vi "timed relay control.vi"(8 "reverse time":u32=350, 9 "start reverse":bool, 10 "start forward":bool, 11 "forward time":u32=350) -> (1 "complete":bool, 3 "output to relay":T1)   [LabVIEW 2016]
uses:
  <vilib>/Rock Robotics/WPI/Relay/WPI_RelayValue.ctl
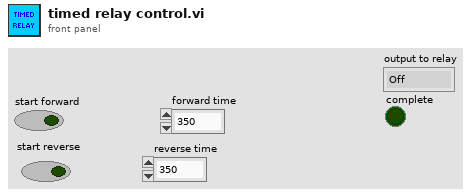
[diagram p1: front panel]
types:
  T1 = typedef "WPI_RelayValue.ctl" = enum16{"Off", "On", "Forward", "Reverse"}
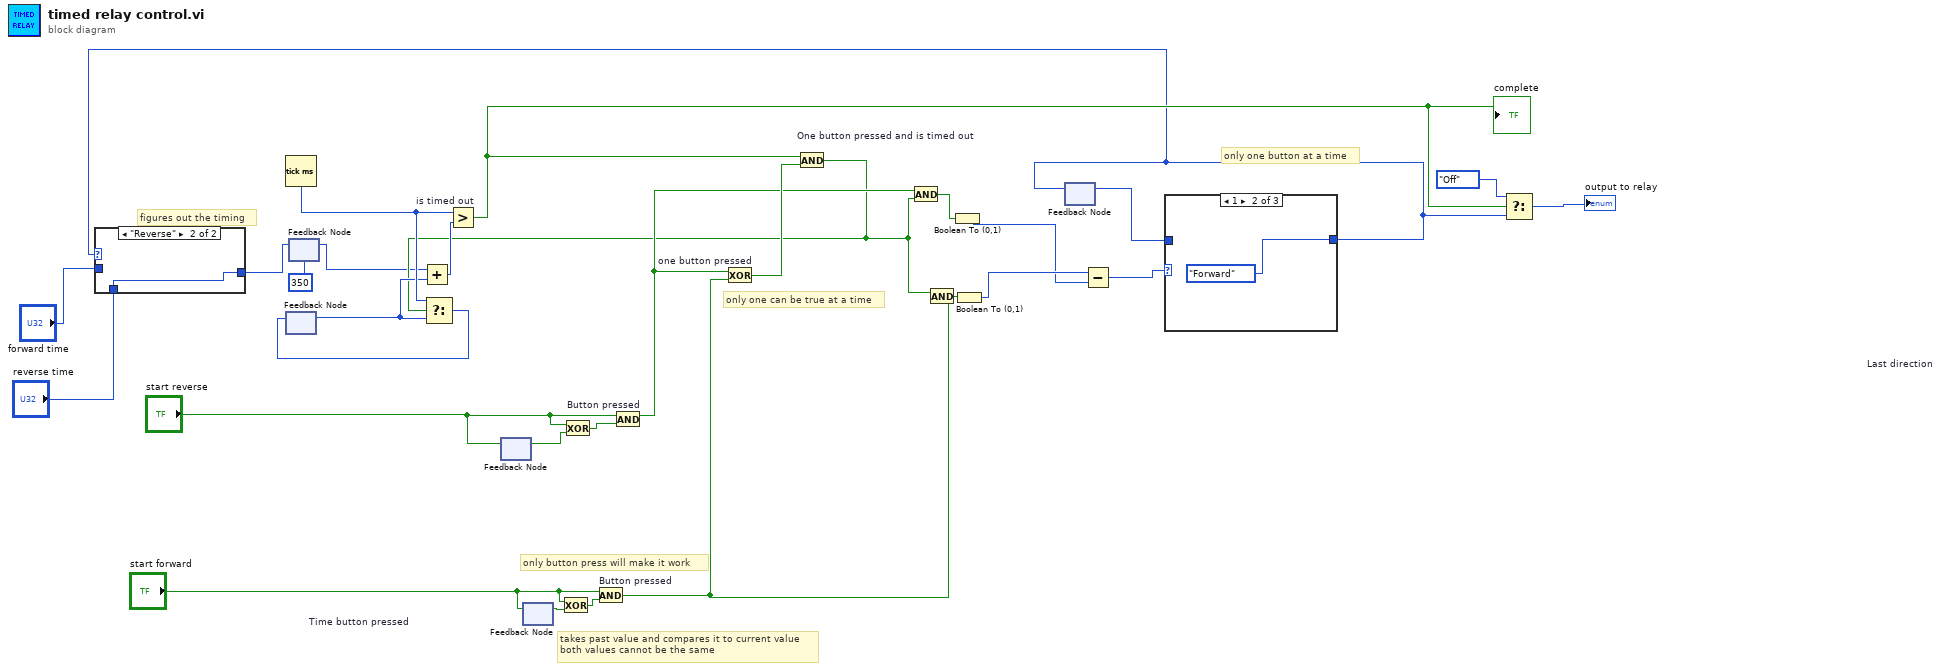
[diagram p0: block diagram]
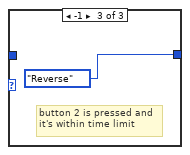
[diagram p4: hidden frame]
diagram:
  # "figures out the timing"
  # "takes past value and compares it to current value\nboth values cannot be the same"
  # "only one button at a time"
  # "only button press will make it work"
  # "only one can be true at a time"
  n1 = Tick Count (ms)() -> (millisecond timer value=w29:u32)
  n2 = feedback #1 "Time button pressed"() -> (w14:u32)  [unwired: 1 in]
  n3 = feedback #2(u32 350 ("y")) -> (w8:u32)
  n4 = Add(x=w8, y=w14) -> (x+y=w27:u32)
  n5 = Greater? "is timed out"(x=w29, y=w27) -> (0:w18:bool)
  "complete" <- w18
  n6 = feedback #3() -> (w25:bool)  [unwired: 1 in]
  n7 = feedback-in #3("start reverse") -> ()
  n8 = feedback #4() -> (w6:bool)  [unwired: 1 in]
  n9 = feedback-in #4("start forward") -> ()
  n10 = Exclusive Or(1:w6, 2:"start forward") -> (0:w26:bool)
  n11 = Exclusive Or(1:w25, 2:"start reverse") -> (0:w24:bool)
  n12 = And "Button pressed"(x="start forward", y=w26) -> (x .and. y?=w13:bool)
  n13 = And "Button pressed"(x="start reverse", y=w24) -> (x .and. y?=w12:bool)
  n14 = Exclusive Or "one button pressed"(1:w13, 2:w12) -> (0:w23:bool)
  n15 = And "One button pressed and is timed out"(x=w18, y=w23) -> (x .and. y?=w11:bool)
  n16 = Select(t=w29, s=w11, f=w14) -> (s? t:f=w28:u32)
  n17 = feedback-in #1(w28) -> ()
  n18 = And(x=w12, y=w11) -> (x .and. y?=w20:bool)
  n19 = And(x=w11, y=w13) -> (x .and. y?=w19:bool)
  n20 = Boolean To (0,1)(Boolean=w20) -> (0, 1=w21:i16)
  n21 = Boolean To (0,1)(Boolean=w19) -> (0, 1=w22:i16)
  n22 = feedback #5 "Last direction"() -> (w16:T1)  [unwired: 1 in]
  n23 = Subtract(x=w22, y=w21) -> (x-y=w15:i16)
  n24 = case shown="1" w15 {
    tunnel: [w30 WPI_RelayValue."Forward" WPI_RelayValue."Reverse" ("RelayValue")] -> w10
    tunnel: w16 -> [w30 _ _]
    frame 0, Default {
    }
    frame 1 {
    }
    frame -1 {
      # "button 2 is pressed and\nit's within time limit"
    }
  }
  n25 = case shown="\"Reverse\"" w10 {
    tunnel: [w33 w34] -> w9
    tunnel: "forward time" -> [w33 _]
    tunnel: "reverse time" -> [_ w34]
    frame "Forward", Default {
    }
    frame "Reverse" {
    }
  }
  n26 = feedback-in #2(w9) -> ()
  n27 = feedback-in #5(w10) -> ()
  n28 = Select(t=WPI_RelayValue."Off" ("RelayValue"), s=w18, f=w10) -> (s? t:f=→"output to relay":T1)
